vi "Test BME680 API.vi"() -> ()   [LabVIEW 2022 SP3]
doc: "BME680 API Tester."
uses:
  <vilib>/Utility/error.llb/DialogType.ctl
  BME680.lvlib
panel:
  out "last error":errorcluster
  in  "Show Diagram on Init":bool
  in  "wait for reply":bool=TRUE
  in  "Show Block Diagram":bool
  in  "X":dbl=1.0
  out "Reply Payload":dbl
  in  "Stop Module":bool
  in  "Start Module":bool
  out "Do Something Count":i32
  in  "Test Do Something Else and Wait for Reply":bool
  in  "Hide Module Panel":bool
  in  "Show Module Panel":bool
  in  "Test Do Something Else":bool
  in  "Test Do Something":bool
  out "Status":string
  out "Module Running?":bool
  # "This VI tests the API for the Module."
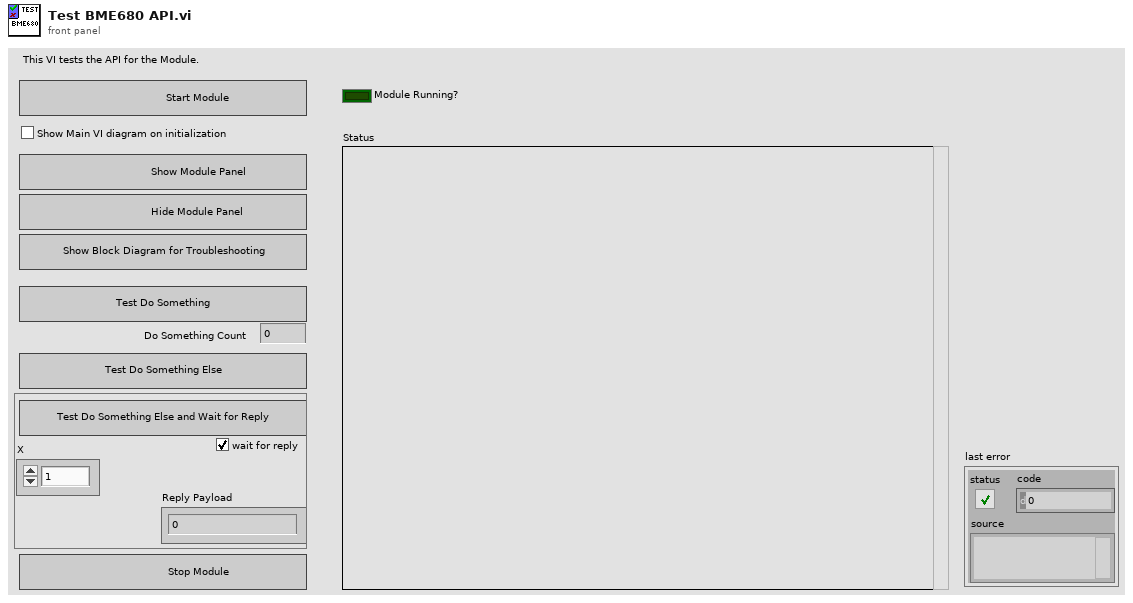
[diagram p1: front panel]
types:
  T1 = typedef "BME680.lvlib/Broadcast Events--cluster.ctl" = cluster{"Module Did Init":refnum<user-event>, "Status Updated":refnum<user-event>, "Error Reported":refnum<user-event>, "Did Something":refnum<user-event>, "Module Did Stop":refnum<user-event>, "Update Module Execution Status":refnum<user-event>}
  T2 = typedef "DialogType.ctl" = u16
  T3 = typedef "BME680.lvlib/Do Something Else and Wait (Reply Payload)--cluster.ctl" = cluster{"Value":dbl, "error":errorcluster}
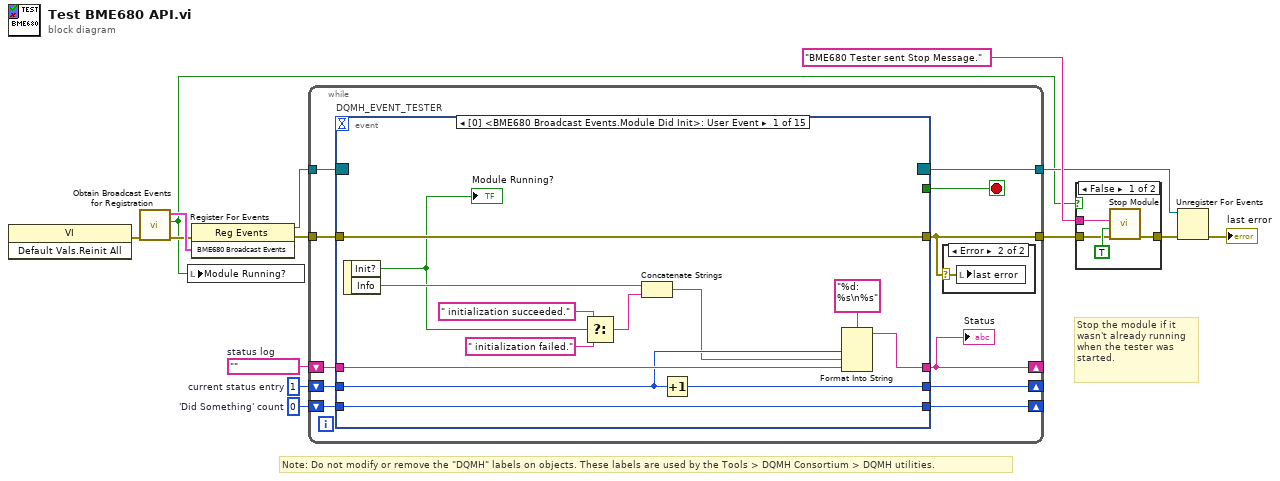
[diagram p0: block diagram]
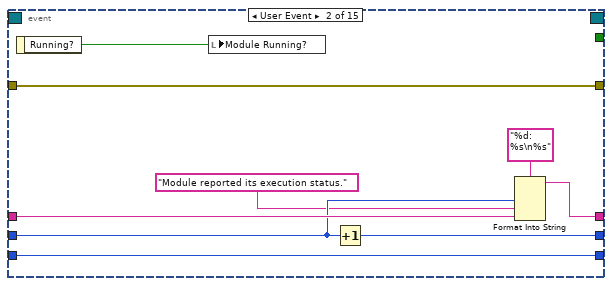
[diagram p4: hidden frame]
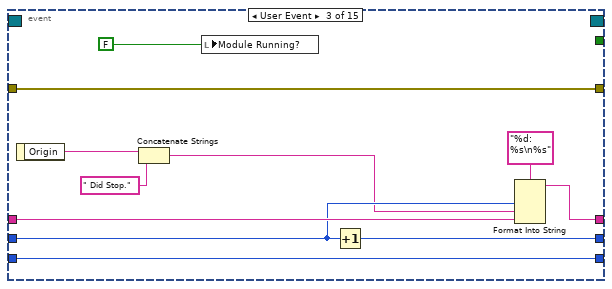
[diagram p5: hidden frame]
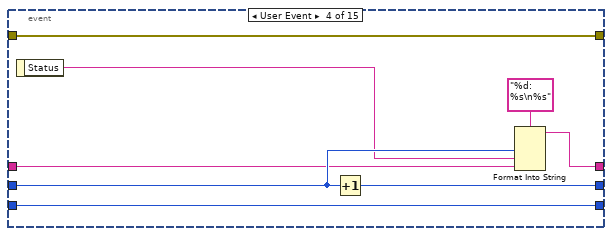
[diagram p6: hidden frame]
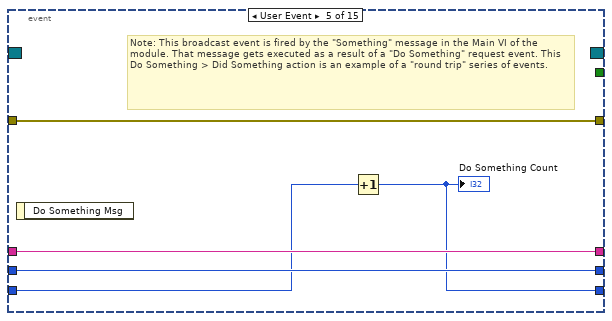
[diagram p7: hidden frame]
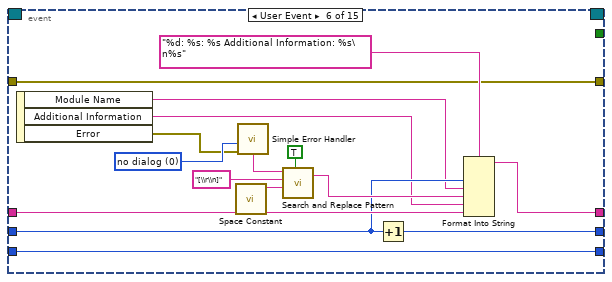
[diagram p8: hidden frame]
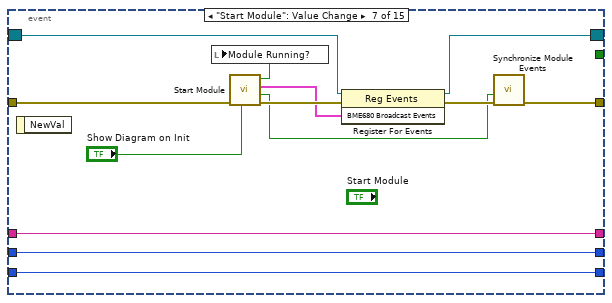
[diagram p9: hidden frame]
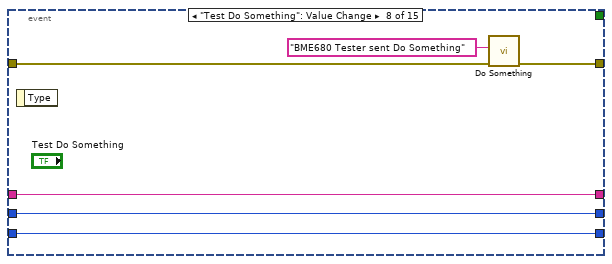
[diagram p10: hidden frame]
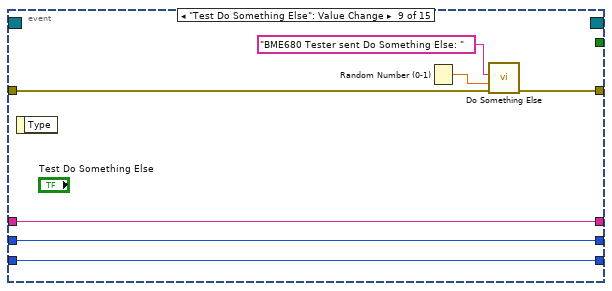
[diagram p11: hidden frame]
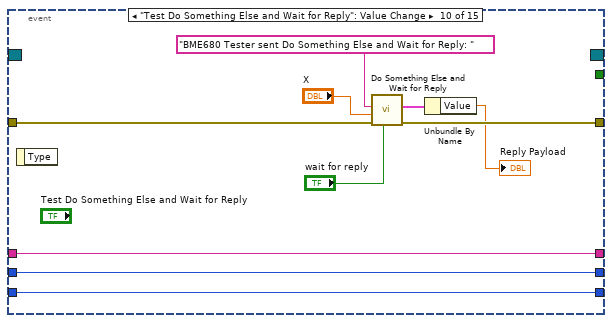
[diagram p12: hidden frame]
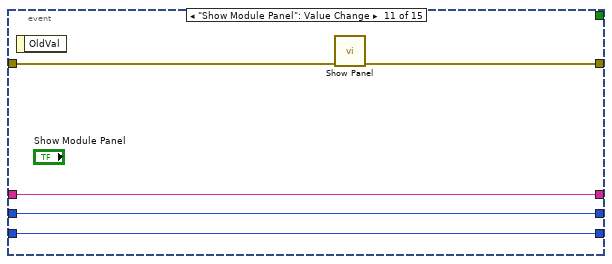
[diagram p13: hidden frame]
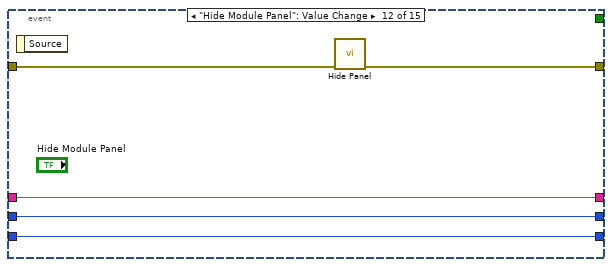
[diagram p14: hidden frame]
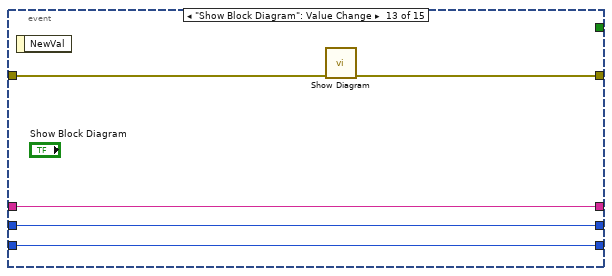
[diagram p15: hidden frame]
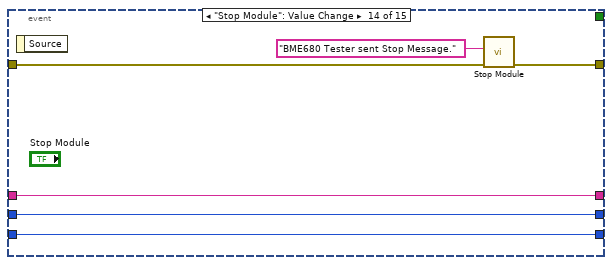
[diagram p16: hidden frame]
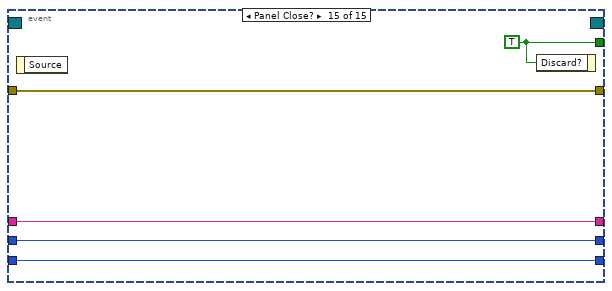
[diagram p17: hidden frame]
diagram:
  w10 = 0  # 'Did Something' count
  w11 = 1  # current status entry
  w12 = ""  # status log
  # "Stop the module if it wasn't already running when the tester was started."
  # "Note: Do not modify or remove the \"DQMH\" labels on objects. These labels are used by the Tools > DQMH Consortium > DQMH utilities."
  n1 = invoke class="VI" method="Default Vals.Reinit All"() -> (error out=w5:errorcluster)  [unwired: 3 in, 2 out]
  n2 = call "Obtain Broadcast Events for Registration.vi"("error in"=w5) -> ("error out"=w4:errorcluster, "Already running?"=w3:bool, "BME680 Broadcast Events"=w8:T1)  [unwired: 8 in]
  n3 = local write "Module Running?"(w3) -> ()
  n4 = register-events(error in=w4, w8) -> (reference out=w7:refnum<event-registration>, error out=w9:errorcluster)  [unwired: 1 in]
  n5 = while {
    tunnel: w7 -> [w25]
    tunnel: [w15] -> w2
    shift-right: [w21] -> _
    shift-left: w12 -> [w23]
    shift-right: [w22] -> _
    shift-left: w11 -> [w24]
    shift-right: [w19] -> _
    shift-left: w10 -> [w20]
    tunnel: w9 -> [w18]
    tunnel: [w17] -> w6
    stop <- w16 stop-if-true
    n6 = event "DQMH_EVENT_TESTER" shown="[0] <BME680 Broadcast Events.Module Did Init>: User Event" {
      selector: w25 -> [_ _ _ _ _ _ w94 _ _ _ _ _ _ _ _]
      dyn-events: [_ _ _ _ _ _ w93 _ _ _ _ _ _ _ _] -> w17
      timeout: _ -> [_ _ _ _ _ _ _ _ _ _ _ _ _ _ _]
      tunnel: [_ _ _ _ _ _ _ _ _ _ _ _ _ _ w150] -> w16
      tunnel: [w39 w41 w49 w60 w68 w76 w92 w107 w114 w124 w129 w134 w135 w142 w146] -> w15
      tunnel: w24 -> [w36 w46 w57 w64 w71 w79 w98 w104 w110 w121 w127 w132 w137 w144 w148]
      tunnel: w23 -> [w37 w47 w58 w63 w72 w80 w99 w105 w111 w122 w128 w133 w138 w145 w149]
      tunnel: [w34 w44 w55 w65 w72 w78 w99 w105 w111 w122 w128 w133 w138 w145 w149] -> w21
      tunnel: [w35 w45 w56 w67 w71 w77 w98 w104 w110 w121 w127 w132 w137 w144 w148] -> w22
      tunnel: w20 -> [w31 w42 w51 w61 w70 w88 w97 w103 w109 w120 w126 w131 w136 w143 w147]
      tunnel: [w31 w42 w51 w61 w69 w88 w97 w103 w109 w120 w126 w131 w136 w143 w147] -> w19
      tunnel: w18 -> [w39 w41 w49 w60 w68 w76 w91 w102 w108 w117 w125 w130 w139 w140 w146]
      event User Event {
        n7 = event-data() -> ("Init?"=w30:bool, "Info"=w33:string)  [unwired: 1 in]
        "Module Running?" <- w30
        n8 = Select(t=" initialization succeeded.", s=w30, f=" initialization failed.") -> (s? t:f=w27:string)
        n9 = Concatenate Strings(w33, w27) -> (w32:string)
        n10 = Increment(x=w36) -> (x+1=w35:i32)
        n11 = Format Into String(format string="%d: %s\n%s", w36, w32, w37) -> (resulting string=w34:string)  [unwired: 2 in, 1 out]
      }
      event User Event {
        n12 = event-data() -> ("Running?"=w40:bool)  [unwired: 1 in]
        n13 = local write "Module Running?"(w40) -> ()
        n14 = Increment(x=w46) -> (x+1=w45:i32)
        n15 = Format Into String(format string="%d: %s\n%s", w46, "Module reported its execution status.", w47) -> (resulting string=w44:string)  [unwired: 2 in, 1 out]
      }
      event User Event {
        n16 = event-data() -> ("Origin"=w54:string)  [unwired: 1 in]
        n17 = Concatenate Strings(w54, " Did Stop.") -> (w53:string)
        n18 = local write "Module Running?"(FALSE ("Module Did Init?")) -> ()
        n19 = Increment(x=w57) -> (x+1=w56:i32)
        n20 = Format Into String(format string="%d: %s\n%s", w57, w53, w58) -> (resulting string=w55:string)  [unwired: 2 in, 1 out]
      }
      event User Event {
        n21 = event-data() -> ("Status"=w62:string)  [unwired: 1 in]
        n22 = Increment(x=w64) -> (x+1=w67:i32)
        n23 = Format Into String(format string="%d: %s\n%s", w64, w62, w63) -> (resulting string=w65:string)  [unwired: 2 in, 1 out]
      }
      event User Event {
        # "Note: This broadcast event is fired by the \"Something\" message in the Main VI of the module. That message gets executed as a result of a \"Do Something\" request event. This Do Something > Did Something action is an example of a \"round trip\" series of events."
        n24 = event-data() -> ()  [unwired: 1 in, 1 out]
        n25 = Increment(x=w70) -> (x+1=w69:i32)
        "Do Something Count" <- w69
      }
      event User Event {
        w81 = T2 0 items=["no dialog", "OK message", "continue or stop message", "OK message + warnings", "continue/stop + warnings"] ("type of dialog (OK msg:1)")
        n26 = event-data() -> ("Module Name"=w75:string, "Additional Information"=w74:string, "Error"=w73:errorcluster)  [unwired: 1 in]
        n27 = call <vilib>:"Space Constant.vi"() -> ("String"=w85:string)
        n28 = call <vilib>:"Simple Error Handler.vi"("type of dialog (OK msg:1)"=w81, "error in (no error)"=w73) -> ("message"=w82:string)  [unwired: 3 in, 4 out]
        n29 = call <vilib>:"Search and Replace Pattern.vi"("string"=w82, "regular expression (\"\")"="[\\r\\n]" ("regular expression (\"\")"), "replace string (\"\")"=w85, "replace all? (F)"=TRUE ("replace all CR/LF with spaces")) -> ("result string"=w83:string)  [unwired: 1 in, 1 out]
        n30 = Increment(x=w79) -> (x+1=w77:i32)
        n31 = Format Into String(format string="%d: %s: %s Additional Information: %s\n%s", w79, w75, w83, w74, w80) -> (resulting string=w78:string)  [unwired: 2 in, 1 out]
      }
      event "Start Module": Value Change {
        n32 = event-data() -> ()  [unwired: 1 in, 1 out]
        n33 = call "Start Module.vi"("Show Main VI Diagram on Init (F)"="Show Diagram on Init", "error in"=w91) -> ("error out"=w100:errorcluster, "Wait for Event Sync?"=w96:bool, "BME680 Broadcast Events"=w95:T1, "Module Was Already Running?"=w90:bool)  [unwired: 6 in]
        n34 = local write "Module Running?"(w90) -> ()
        n35 = register-events(reference=w94, error in=w100, w95) -> (reference out=w93:refnum<event-registration>, error out=w101:errorcluster)
        n36 = call "Synchronize Module Events.vi"("error in"=w101, "Wait for Event Sync?"=w96) -> ("error out"=w92:errorcluster)  [unwired: 9 in]
      }
      event "Test Do Something": Value Change {
        n37 = event-data() -> ()  [unwired: 1 in, 1 out]
        n38 = call "Do Something.vi"("error in"=w102, "Do Something Message"="BME680 Tester sent Do Something") -> ("error out"=w107:errorcluster)  [unwired: 9 in]
      }
      event "Test Do Something Else": Value Change {
        n39 = event-data() -> ()  [unwired: 1 in, 1 out]
        n40 = Random Number (0-1)() -> (number: 0 to 1=w112:dbl)
        n41 = call "Do Something Else.vi"("error in"=w108, "X"=w112, "Do Something Else Message"="BME680 Tester sent Do Something Else: " ("Do Something Message")) -> ("error out"=w114:errorcluster)  [unwired: 8 in]
      }
      event "Test Do Something Else and Wait for Reply": Value Change {
        n42 = event-data() -> ()  [unwired: 1 in, 1 out]
        n43 = call "Do Something Else and Wait for Reply.vi"("wait for reply (T)"="wait for reply", "error in"=w117, "X"="X", "Do Something Else Message"="BME680 Tester sent Do Something Else and Wait for Reply: " ("Do Something Message")) -> ("error out"=w124:errorcluster, "Reply Payload"=w119:T3)  [unwired: 5 in, 1 out]
        n44 = Unbundle By Name(w119) -> ("Value"=→"Reply Payload":dbl)
      }
      event "Show Module Panel": Value Change {
        n45 = event-data() -> ()  [unwired: 1 in, 1 out]
        n46 = call "Show Panel.vi"("error in"=w125) -> ("error out"=w129:errorcluster)  [unwired: 10 in]
      }
      event "Hide Module Panel": Value Change {
        n47 = event-data() -> ()  [unwired: 1 in, 1 out]
        n48 = call "Hide Panel.vi"("error in"=w130) -> ("error out"=w134:errorcluster)  [unwired: 10 in]
      }
      event "Show Block Diagram": Value Change {
        n49 = event-data() -> ()  [unwired: 1 in, 1 out]
        n50 = call "Show Diagram.vi"("error in"=w139) -> ("error out"=w135:errorcluster)  [unwired: 10 in]
      }
      event "Stop Module": Value Change {
        n51 = event-data() -> ()  [unwired: 1 in, 1 out]
        n52 = call "Stop Module.vi"("error in"=w140, "Origin"="BME680 Tester sent Stop Message.") -> ("error out"=w142:errorcluster)  [unwired: 9 in]
      }
      event Panel Close? {
        w150 = TRUE ("Discard?")
        n53 = event-data() -> ()  [unwired: 1 in, 1 out]
        n54 = event-data("Discard?"=w150) -> ()  [unwired: 1 in, 1 out]
      }
    }
    "Status" <- w21
    n55 = case shown="Error" w15 {
      selector: w15 -> [_ w26]
      frame No Error {
      }
      frame Error {
        n56 = local write "last error"(w26) -> ()
      }
    }
  }
  n57 = case shown="False" w3 {
    tunnel: [w154 w155] -> w14
    tunnel: "BME680 Tester sent Stop Message." ("Origin") -> [w153 _]
    tunnel: w2 -> [w151 w155]
    frame False {
      n58 = call "Stop Module.vi"("error in"=w151, "Wait for Module to Stop? (F)"=TRUE ("Wait for Module to stop?"), "Origin"=w153) -> ("error out"=w154:errorcluster)  [unwired: 8 in]
    }
    frame True {
    }
  }
  n59 = Unregister For Events(event registration refnum=w6, error in=w14) -> (error out=→"last error":errorcluster)
